vi "Shoot Control Loop.vi"() -> ()   [LabVIEW 2019]
uses:
  Calculations or utilities/Is command done typedef.ctl
  <vilib>/Rock Robotics/WPI/ThirdParty/Phoenix-LabVIEW/Motor Controller/Controls/CTRE_Phoenix_MotorControl_ControlMode.ctl
  Shoot Global.vi
  <vilib>/Rock Robotics/WPI/ThirdParty/Phoenix-LabVIEW/Motor Controller/Get/CTRE_Phoenix_MotorController_GetSelectedSensorData.vi
panel:
  out "Shooter Velocity (RPM)":dbl(graph)
  in  "Acceptable Error (RPM)":dbl=20.0
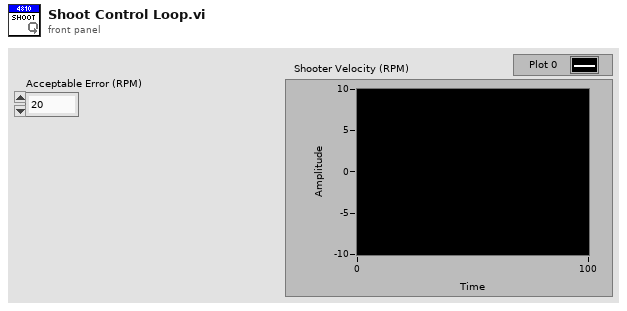
[diagram p1: front panel]
types:
  T1 = typedef "WPI_MotorControlDeviceRef.ctl" = cluster{"DeviceStatus":errorcluster, "Type":T2, "PWM":cluster{"PWM Channel":T3, "DeadBand":T4}, "CAN":cluster{"Device Number":u8, "SetOutput VI Ref":variant, "GetOutput VI Ref":variant, "Enable VI Ref":variant, "Disable VI Ref":variant, "Data":variant}, "Invert":bool, "DIO PWM":cluster{"PWM \"Enable\" Channel":T3, "DIOChannel":T5, "PWM Rate":dbl}}
  T2 = typedef "WPI_MotorControlType.ctl" = enum16{"PWM", "CAN", "DIO PWM"}
  T3 = typedef "FPGA_DIOPWMChannel.ctl" = enum8{"PWM 0", "PWM 1", "PWM 2", "PWM 3", "PWM 4", "PWM 5", "PWM 6", "PWM 7", "PWM 8", "PWM 9", "PWM MXP 0", "PWM MXP 1", "PWM MXP 2", "PWM MXP 3", "PWM MXP 4", "PWM MXP 5", "PWM MXP 6", "PWM MXP 7", "PWM MXP 8", "PWM MXP 9", "Invalid"}
  T4 = typedef "WPI_PWMDeadband.ctl" = cluster{"Name":string, "maxPositivePwm":i32, "minPositivePwm":i32, "centerPwm":i32, "maxNegativePwm":i32, "minNegativePwm":i32, "angularRange":u16}
  T5 = typedef "FPGA_DIOChannel.ctl" = enum8{"DIO 0", "DIO 1", "DIO 2", "DIO 3", "DIO 4", "DIO 5", "DIO 6", "DIO 7", "DIO 8", "DIO 9", "DIO MXP 0", "DIO MXP 1", "DIO MXP 2", "DIO MXP 3", "DIO MXP 4", "DIO MXP 5", "DIO MXP 6", "DIO MXP 7", "DIO MXP 8", "DIO MXP 9", "DIO MXP 10", "DIO MXP 11", "DIO MXP 12", "DIO MXP 13", "DIO MXP 14", "DIO MXP 15", "SPI Port CS1", "SPI Port CS2", "SPI Port CS3", "SPI Port MISO", "SPI Port MOSI", "Invalid"}
  T6 = typedef "Is command done typedef.ctl" = cluster{"Done?":bool, "Timestamp [ms]":dbl}
  T7 = typedef "Shooter Command Type Def.ctl" = cluster{"Shooter Mode":T8, "Throttle (%)/ Vision-based\nSetpoint (RPM)":dbl, "Shooter Preset speeds (RPM)":T9, "Timestamp (ms)":dbl}
  T8 = typedef "Shooter Mode Type Def.ctl" = enum16{"Disabled", "Raw Throttle", "Preset Velocity Control", "Vision-based Velocity Control"}
  T9 = typedef "Shooter Preset speeds Type Def.ctl" = enum16{"Target Zone", "Initiation Line", "Close end of Trench Run", "Control Panel"}
  T10 = typedef "CTRE_Phoenix_MotorControl_ControlMode.ctl" = u16
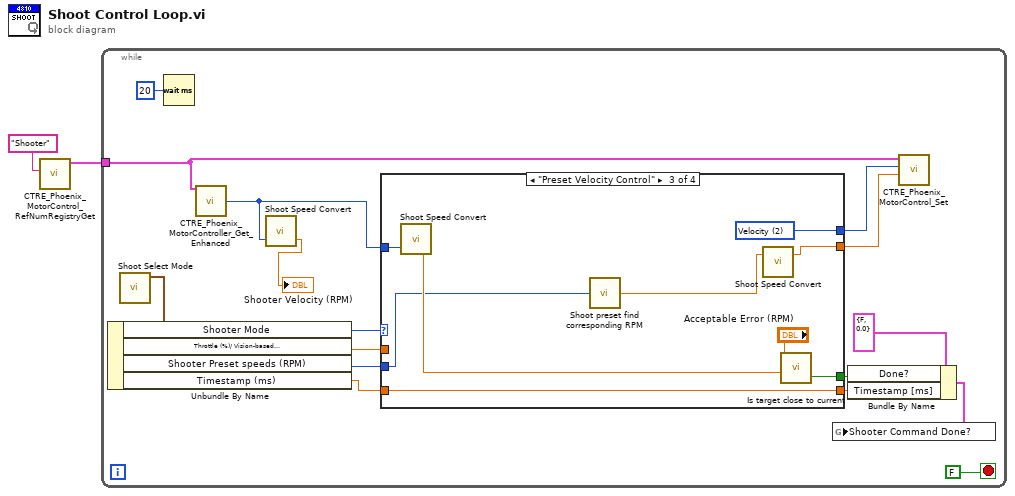
[diagram p0: block diagram]
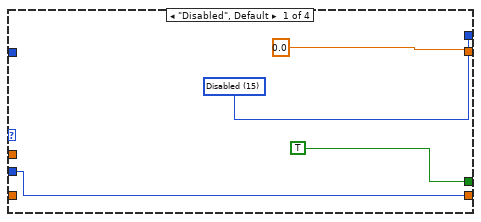
[diagram p2: hidden frame]
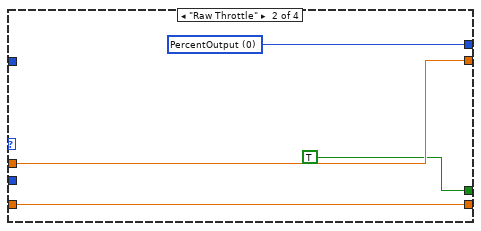
[diagram p3: hidden frame]
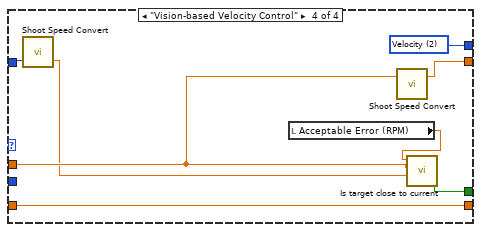
[diagram p4: hidden frame]
diagram:
  n1 = call <vilib>:"CTRE_Phoenix_MotorControl_RefNumRegistryGet.vi"("refnum name"="Shooter") -> ("PhoenixMotorControlDevRef"=w1:T1)  [unwired: 9 in, 1 out]
  n2 = while {
    tunnel: w1 -> [w8]
    stop <- FALSE stop-if-true
    n3 = call "Shoot Select Mode.vi"() -> ("Auton Shooter Command"=w16:T7)  [unwired: 11 in]
    n4 = Unbundle By Name(w16) -> ("Shooter Mode"=w15:T8, "Throttle (%)/ Vision-based\nSetpoint (RPM)"=w12:dbl, "Shooter Preset speeds (RPM)"=w11:T9, "Timestamp (ms)"=w6:dbl)
    n5 = Wait (ms)(milliseconds to wait=u32 20) -> ()  [unwired: 1 out]
    n6 = call-poly <vilib>:"CTRE_Phoenix_MotorController_Get_Enhanced.vi"("PhoenixMotorControlDevRef"=w8) -> ("Velocity (Raw Sensor Units per 100 ms)"=w4:i32)  [unwired: 11 in, 3 out]
    n7 = call "Shoot Speed Convert.vi"("Shooter speed in (u/100ms)"=w4) -> ("Shooter Speed out (RPM)"=→"Shooter Velocity (RPM)":dbl)  [unwired: 1 in, 1 out]
    n8 = case shown="\"Preset Velocity Control\"" w15 {
      tunnel: [w22 w26 w35 w43] -> w14
      tunnel: [0.0 ("Shoot") w25 w29 w42] -> w13
      tunnel: w12 -> [_ w25 _ w38]
      tunnel: w11 -> [w20 _ w28 _]
      tunnel: [TRUE ("Done?") TRUE ("Done?") w33 w40] -> w9
      tunnel: w4 -> [_ _ w31 w41]
      tunnel: w6 -> [_ w23 w32 w36]
      tunnel: [w20 w23 w32 w36] -> w5
      frame "Disabled", Default {
        w22 = T10 15 items=["PercentOutput"=0, "Position"=1, "Velocity"=2, "Current"=3, "Follower"=5, "MotionProfile"=6, "MotionMagic"=7, "MotionProfileArc"=10, "Disabled"=15] ("Control Mode")
      }
      frame "Raw Throttle" {
        w26 = T10 0 items=["PercentOutput"=0, "Position"=1, "Velocity"=2, "Current"=3, "Follower"=5, "MotionProfile"=6, "MotionMagic"=7, "MotionProfileArc"=10, "Disabled"=15] ("Control Mode")
      }
      frame "Preset Velocity Control" {
        w35 = T10 2 items=["PercentOutput"=0, "Position"=1, "Velocity"=2, "Current"=3, "Follower"=5, "MotionProfile"=6, "MotionMagic"=7, "MotionProfileArc"=10, "Disabled"=15] ("Control Mode")
        n9 = call "Shoot Speed Convert.vi"("Shooter speed in (u/100ms)"=w31) -> ("Shooter Speed out (RPM)"=w30:dbl)  [unwired: 1 in, 1 out]
        n10 = call "Shoot preset find corresponding RPM.vi"("Shooter Preset speeds (RPM)"=w28) -> ("Shooter Speed (RPM)"=w27:dbl)
        n11 = call "Shoot Speed Convert.vi"("Shooter speed in (RPM)"=w27) -> ("Shooter Speed out (u/100ms)"=w29:dbl)  [unwired: 1 in, 1 out]
        n12 = call "Is target close to current.vi"("Current Position"=w30, "Acceptable Error"="Acceptable Error (RPM)") -> ("Acceptable"=w33:bool)  [unwired: 9 in]
      }
      frame "Vision-based Velocity Control" {
        w43 = T10 2 items=["PercentOutput"=0, "Position"=1, "Velocity"=2, "Current"=3, "Follower"=5, "MotionProfile"=6, "MotionMagic"=7, "MotionProfileArc"=10, "Disabled"=15] ("Control Mode")
        n13 = call "Shoot Speed Convert.vi"("Shooter speed in (u/100ms)"=w41) -> ("Shooter Speed out (RPM)"=w37:dbl)  [unwired: 1 in, 1 out]
        n14 = local read "Acceptable Error (RPM)"() -> (w39:dbl)
        n15 = call "Shoot Speed Convert.vi"("Shooter speed in (RPM)"=w38) -> ("Shooter Speed out (u/100ms)"=w42:dbl)  [unwired: 1 in, 1 out]
        n16 = call "Is target close to current.vi"("Current Position"=w37, "Target Position"=w38, "Acceptable Error"=w39) -> ("Acceptable"=w40:bool)  [unwired: 8 in]
      }
    }
    n17 = Bundle By Name(cluster=T6 {"Done?"=FALSE, "Timestamp [ms]"=0.0} ("Command Done?"), "Done?"=w9, "Timestamp [ms]"=w5) -> (w7:T6)
    n18 = global write "Shoot Global.vi" "Shooter Command Done?"(w7) -> ()
    n19 = call <vilib>:"CTRE_Phoenix_MotorControl_Set.vi"("Output"=w13, "Control Mode"=w14, "PhoenixMotorControlDevRef"=w8) -> ()  [unwired: 7 in, 2 out]
  }
